vi "ForLoop to Code.vi"(8 "error in":errorcluster, 11 "GObj Refnum":refnum<vi>) -> (0 "error out":errorcluster, 2 "WhileLoop code chunks":T1, 3 "terminals info":T2)   [LabVIEW 2014]
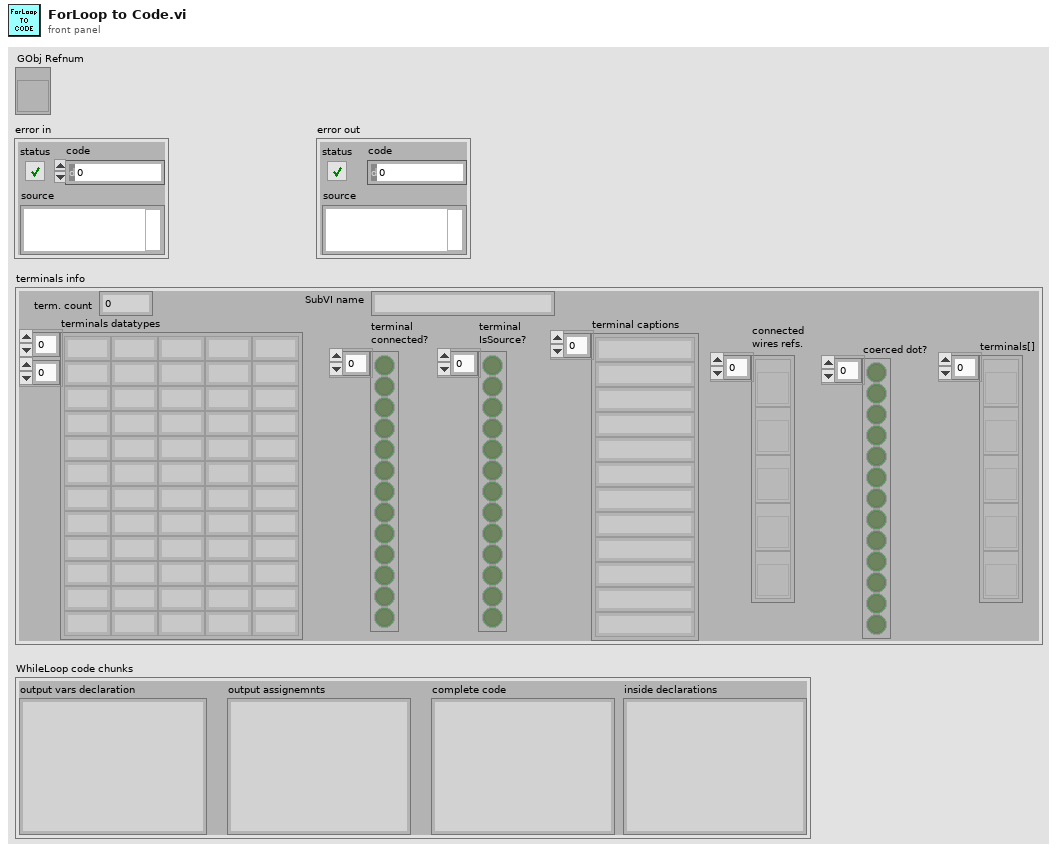
[diagram p1: front panel]
types:
  T1 = cluster{"output vars declaration":string, "output assignemnts":string, "complete code":string, "inside declarations":string}
  T2 = cluster{"terminals datatypes":string[][], "terminal\nconnected?":bool[], "terminal captions":string[], "term. count":i32, "terminal\nIsSource?":bool[], "SubVI name":string, "connected\nwires refs.":refnum<vi>[], "coerced dot?":bool[], "terminals[]":refnum<vi>[]}
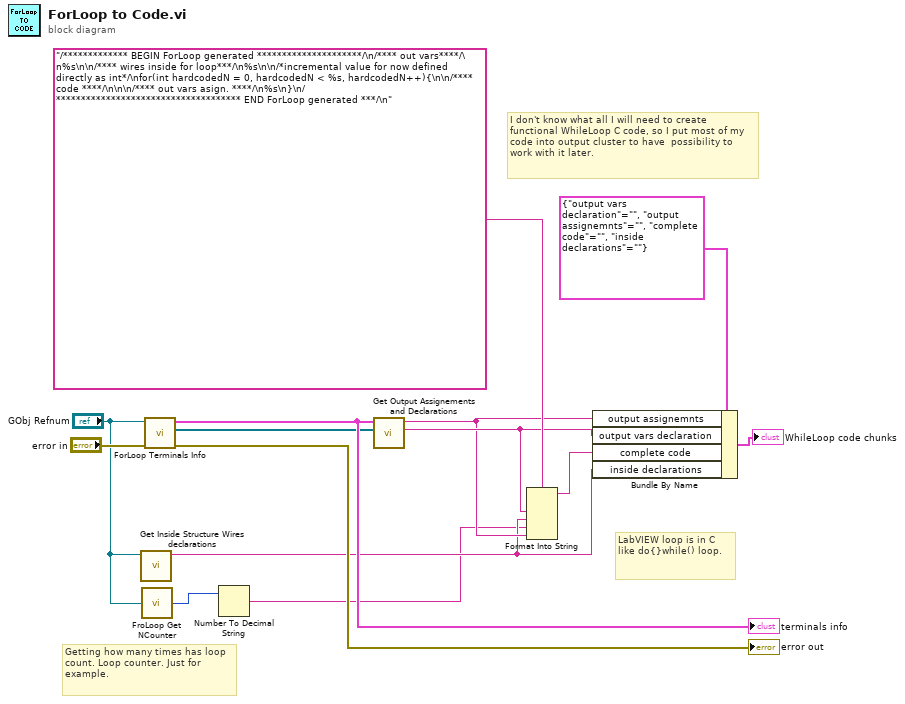
[diagram p0: block diagram]
diagram:
  # "Getting how many times has loop count. Loop counter. Just for example."
  # "I don't know what all I will need to create functional WhileLoop C code, so I put most of my code into output cluster to have  possibility to work with it later."
  # "LabVIEW loop is in C like do{}while() loop."
  n1 = call "Get Inside Structure Wires declarations.vi"("GObject in"="GObj Refnum") -> ("structure inside wires C declarations"=w2:string)  [unwired: 10 in]
  n2 = call "FroLoop Get NCounter.vi"("reference"="GObj Refnum") -> ("ForLoopN"=w3:i32)
  n3 = call "ForLoop Terminals Info.vi"("error in"="error in", "GObj Refnum"="GObj Refnum") -> ("error out"=→"error out":errorcluster, "Terminals[]"=w11:refnum<vi>[], "output cluster"=w12:T2)  [unwired: 7 in]
  "terminals info" <- w12
  n4 = Number To Decimal String(number=w3) -> (decimal integer string=w1:string)  [unwired: 1 in]
  n5 = call "Get Output Assignements and Declarations.vi"("structure terminals[]"=w11, "output cluster"=w12) -> ("output declarations"=w6:string, "outuput assignements"=w5:string)  [unwired: 7 in, 1 out]
  n6 = Format Into String(format string="/************* BEGIN ForLoop generated *********************/\n/**** out vars****/\n%s\n\n/**** wires inside for loop***/\n%s\n\n/*incremental value for now defined directly as int*/\nfor(int hardcodedN = 0, hardcodedN < %s, hardcodedN++){\n\n/**** code ****/\n\n\n/**** out vars asign. ****/\n%s\n}\n/************************************* END ForLoop generated ***/\n", w6, w2, w1, w5) -> (resulting string=w7:string)  [unwired: 2 in, 1 out]
  n7 = Bundle By Name(cluster=T1 {"output vars declaration"="", "output assignemnts"="", "complete code"="", "inside declarations"=""}, "output assignemnts"=w5, "output vars declaration"=w6, "complete code"=w7, "inside declarations"=w2) -> (→"WhileLoop code chunks":T1)
